vi "sendCommand.vi"(6 "Wait for response (T)":bool=TRUE, 8 "error in (no error)":errorcluster, 9 "timeout (ms)":i32=-1, 10 "command":string, 11 "LabVIEW-Python-Interface in":refnum<class "PyLVi.lvclass">) -> (0 "error out":errorcluster, 1 "timeout?":bool, 2 "data":string, 3 "LabVIEW-Python-Interface out":refnum<class "PyLVi.lvclass">)   [LabVIEW 2016, in "PyLVi.lvlib" / "PyLVi.lvclass"]
doc: "Sends a command via the ZMQ socket.\nIf \"Wait for response\" is False, the function will immediately return after sending. The data string will then be empty.\nIn case \"Wait for response\" is True, the function will block until a message is received on the socket."
uses:
  PyLVi.lvclass
  PyLVi.lvclass/PyLVi.ctl
  <vilib>/addons/zeromq/zmq_socket.lvclass
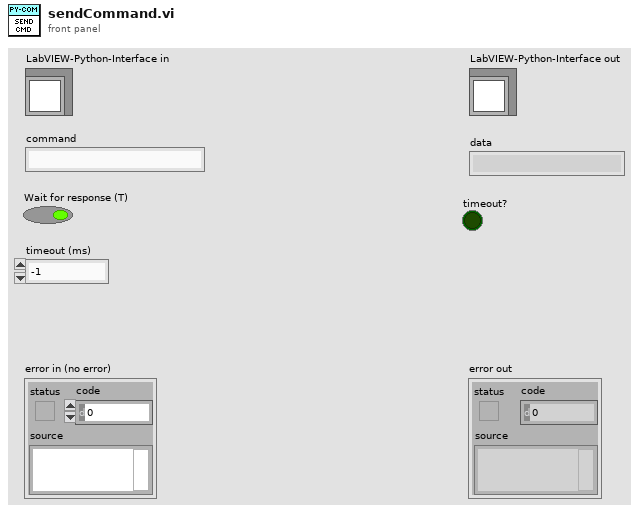
[diagram p1: front panel]
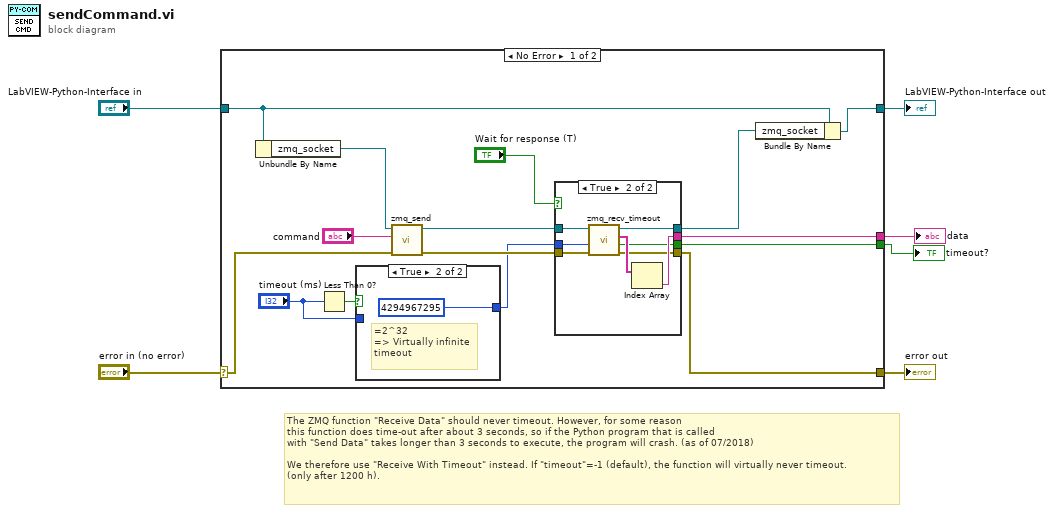
[diagram p0: block diagram]
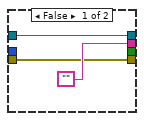
[diagram p3: hidden frame]
diagram:
  # "The ZMQ function \"Receive Data\" should never timeout. However, for some reason\nthis function does time-out after about 3 seconds, so if the Python program that is called\nwith \"Send Data\" takes longer than 3 seconds to execute, the program will crash. (as of 07/2018)\n\nWe therefore use \"Receive With Timeout\" instead. If \"timeout\"=-1 (default), the function will virtually never timeout.\n(only after 1200 h)."
  n1 = case shown="No Error" "error in (no error)" {
    selector: "error in (no error)" -> [w17 w36]
    tunnel: [w11 w36] -> w5
    tunnel: [w18 w35] -> w3
    tunnel: "LabVIEW-Python-Interface in" -> [w19 w35]
    tunnel: [w12 _] -> w2
    tunnel: [w7 _] -> w1
    frame No Error {
      n2 = Unbundle By Name(w19) -> ("zmq_socket"=w20:refnum<class "zmq_socket.lvclass">)
      n3 = Less Than 0?(x="timeout (ms)") -> (x < 0?=w10:bool)
      n4 = case shown="True" w10 {
        tunnel: [w22 u32 4294967295 ("timeout (ms)")] -> w8
        tunnel: "timeout (ms)" -> [w22 _]
        frame False {
        }
        frame True {
          # "=2^32\n=> Virtually infinite\ntimeout"
        }
      }
      n5 = call <vilib>:"zmq_send.vi"("error in"=w17, "data"="command", "socket in"=w20) -> ("error out"=w14:errorcluster, "socket out"=w15:refnum<class "zmq_socket.lvclass">)  [unwired: 4 in]
      n6 = case shown="True" "Wait for response (T)" {
        tunnel: [w25 w32] -> w13
        tunnel: ["" w30] -> w12
        tunnel: [w24 w29] -> w11
        tunnel: w15 -> [w25 w34]
        tunnel: w14 -> [w24 w33]
        tunnel: [_ w28] -> w7
        tunnel: w8 -> [_ w27]
        frame False {
        }
        frame True {
          n7 = call <vilib>:"zmq_recv_timeout.vi"("error in"=w33, "timeout (ms)"=w27, "socket in"=w34) -> ("error out"=w29:errorcluster, "timeout?"=w28:bool, "parts"=w31:string[], "socket out"=w32:refnum<class "zmq_socket.lvclass">)  [unwired: 1 in]
          n8 = Index Array(array=w31) -> (element=w30:string)  [unwired: 1 in]
        }
      }
      n9 = Bundle By Name(cluster=w19, "zmq_socket"=w13) -> (w18:refnum<class "PyLVi.lvclass">)
    }
    frame Error {
    }
  }
  "error out" <- w5
  "LabVIEW-Python-Interface out" <- w3
  "data" <- w2
  "timeout?" <- w1
